vi "Pre-Arm.vi"(8 "error in (no error)":errorcluster, 11 "Red Pitaya Digitizer in":refnum<class "Red Pitaya Digitizer.lvclass">) -> (0 "error out":errorcluster, 3 "Red Pitaya Digitizer out":refnum<class "Red Pitaya Digitizer.lvclass">)   [LabVIEW 2024, in "Red Pitaya Digitizer.lvclass"]
uses:
  Red Pitaya Digitizer.lvclass
  <vilib>/Utility/error.llb/Error Cluster From Error Code.vi
  RP Core/RP Instrument/RP Instrument.lvclass
  <vilib>/ErrorRing/Error Ring.xnode
  Instruments/Pulse Driver/Lockin Digitizer Driver/Lockin Digitizer Driver.lvclass
  File/File Class/File.lvclass
panel:
  out "All channels present":bool
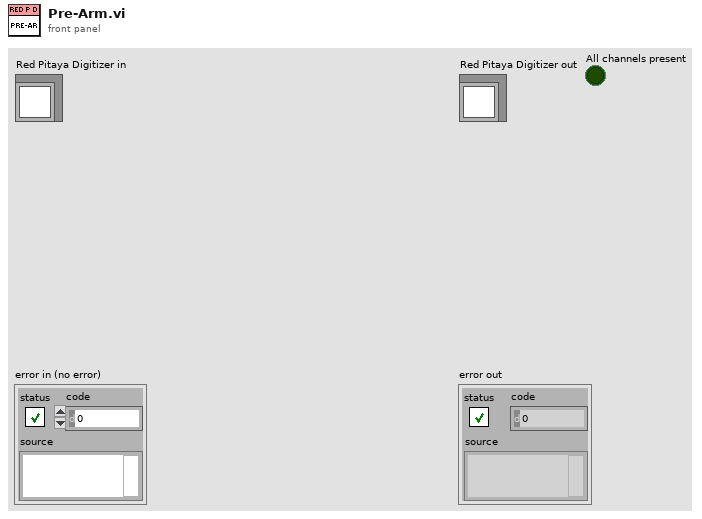
[diagram p1: front panel]
types:
  T1 = typedef "Pusle Driver Configuration.ctl" = cluster{"Post-trigger delay":dbl, "Post-trigger duration":dbl, "Rate":dbl, "Ranges":dbl[], "Re-name channels":string[], "Active channels":string, "External clock":bool}
  T2 = map{i32, cluster{"Module":i32, "Local channel":i32}}
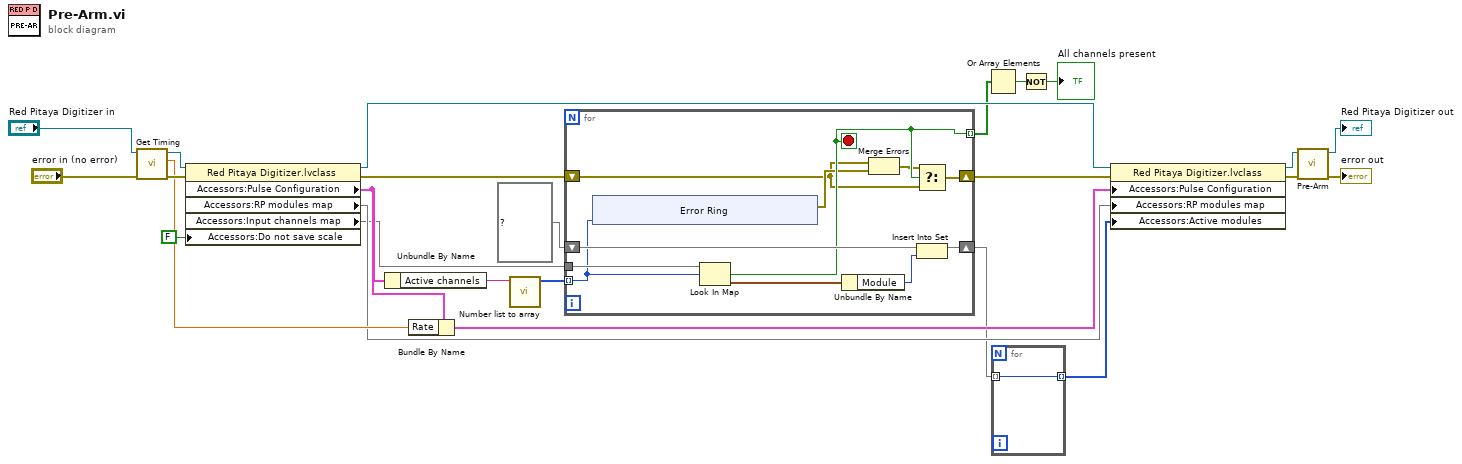
[diagram p0: block diagram]
diagram:
  n1 = call-dynamic "Get Timing.vi"("error in (no error)"="error in (no error)", "Red Pitaya Digitizer in"="Red Pitaya Digitizer in") -> ("error out"=w17:errorcluster, "Rate"=w14:dbl, "Red Pitaya Digitizer out"=w18:refnum<class "Red Pitaya Digitizer.lvclass">)  [unwired: 6 in, 1 out]
  n2 = property class="Red Pitaya Digitizer.lvclass"(reference=w18, error in=w17, "Accessors:Do not save scale"=FALSE ("Do not save scale")) -> (reference out=w15:refnum<class "Red Pitaya Digitizer.lvclass">, error out=w3:errorcluster, "Accessors:Pulse Configuration"=w19:T1, "Accessors:RP modules map "=w12:map{i32, refnum<class "RP Instrument.lvclass">}, "Accessors:Input channels map"=w10:T2)
  n3 = Unbundle By Name(w19) -> ("Active channels"=w13:string)
  n4 = Bundle By Name(cluster=w19, "Rate"=w14) -> (w16:T1)
  n5 = call "Number list to array.vi"("Number list"=w13) -> ("Number list array"=w11:i32[])  [unwired: 7 in, 3 out]
  n6 = for {
    tunnel: w11 -> [w26] mode=indexing
    tunnel: w10 -> [w36]
    tunnel: [w31] -> w9 mode=indexing
    shift-right: [w32] -> w5
    shift-left: set{i32} {} ("set") -> [w35]
    shift-right: [w27] -> w2
    shift-left: w3 -> [w28]
    stop <- w31 stop-if-true
    n7 = xnode "Error Ring"("parameter 0"=w26) -> ("error out"=w30:errorcluster)
    n8 = Look In Map(map=w36, key=w26) -> (key not found?=w31:bool, value=w34:cluster{"Module":i32, "Local channel":i32})  [unwired: 1 in]
    n9 = Unbundle By Name(w34) -> ("Module"=w33:i32)
    n10 = Merge Errors(w28, w30) -> (w29:errorcluster)
    n11 = Select(t=w29, s=w31, f=w28) -> (s? t:f=w27:errorcluster)
    n12 = Insert Into Set(10:w33, 11:w35) -> (3:w32:set{i32})  [unwired: 1 out]
  }
  n13 = Or Array Elements(Boolean array=w9) -> (logical OR=w8:bool)
  n14 = for {
    tunnel: w5 -> [w44] mode=indexing
    tunnel: [w44] -> w4 mode=indexing
  }
  n15 = Not(x=w8) -> (.not. x?=→"All channels present":bool)
  n16 = property class="Red Pitaya Digitizer.lvclass"(reference=w15, error in=w2, "Accessors:Pulse Configuration"=w16, "Accessors:RP modules map "=w12, "Accessors:Active modules"=w4) -> (reference out=w21:refnum<class "Red Pitaya Digitizer.lvclass">, error out=w20:errorcluster)
  n17 = call-parent "Pre-Arm.vi"("error in (no error)"=w20, "Lockin Digitizer Driver in"=w21) -> ("error out"=→"error out":errorcluster, "Lockin Digitizer Driver out"=→"Red Pitaya Digitizer out":refnum<class "Red Pitaya Digitizer.lvclass">)  [unwired: 8 in]
